vi "uuid_myo.vi"(11 "MYO  UUID (16bits)":string="0001") -> (3 "full UUID":string)   [LabVIEW 2013]
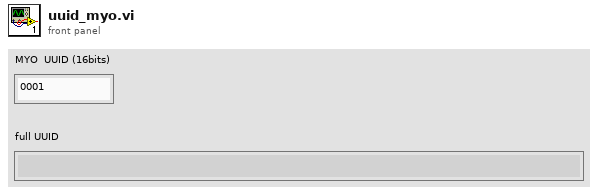
[diagram p1: front panel]
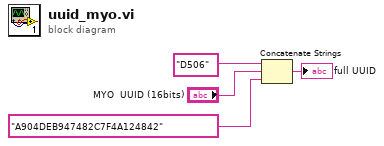
[diagram p0: block diagram]
diagram:
  n1 = Concatenate Strings("D506" ("Characteristic UUID"), "MYO  UUID (16bits)", "A904DEB947482C7F4A124842" ("Characteristic UUID")) -> (→"full UUID":string)
